vi "Update Right Position.vi"(10 "RPosition":dbl, 11 "drive in":refnum<class "drive.lvclass">) -> (3 "drive out":refnum<class "drive.lvclass">)   [LabVIEW 2015, in "drive.lvclass"]
uses:
  drive.lvclass
  drive.lvclass/drive.ctl
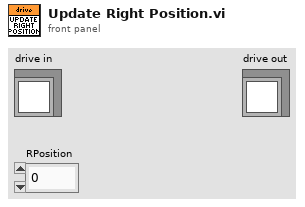
[diagram p1: front panel]
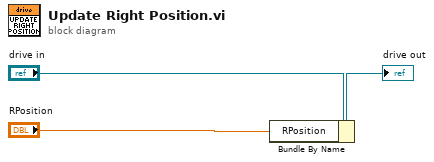
[diagram p0: block diagram]
diagram:
  n1 = Bundle By Name(cluster="drive in", "RPosition"="RPosition") -> (→"drive out":refnum<class "drive.lvclass">)
